vi "PDE_Check Tridiag Solver Platform.vi"(8 "error in (no error)":errorcluster) -> (0 "error out":errorcluster)   [LabVIEW 2017, in "NI_PDE.lvlib"]
uses:
  <vilib>/gmath/NI_PDE.lvlib
  <vilib>/Analysis/NI_AALPro.lvlib
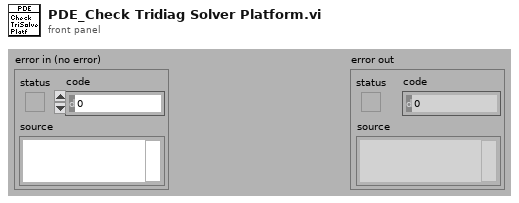
[diagram p1: front panel]
types:
  T1 = cluster{"Diagonal":dbl[], "Super Diagonal":dbl[], "2nd Super Diagonal":dbl[]}
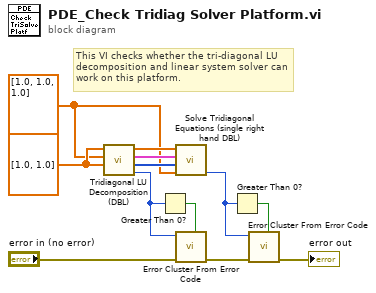
[diagram p0: block diagram]
diagram:
  w7 = dbl[] [1.0, 1.0, 1.0] ("Sub Diagonal")
  w12 = dbl[] [1.0, 1.0] ("Sub Diagonal")
  # "This VI checks whether the tri-diagonal LU decomposition and linear system solver can work on this platform."
  n1 = call <vilib>:"Tridiagonal LU Decomposition (DBL).vi"("Super Diagonal"=w12, "Diagonal"=w7, "Sub Diagonal"=w12) -> ("error"=w4:i32, "Pivot"=w8:i32[], "U"=w9:T1, "L"=w10:dbl[])  [unwired: 5 out]
  n2 = Greater Than 0?(x=w4) -> (x > 0?=w6:bool)
  n3 = call <vilib>:"Solve Tridiagonal Equations (single right hand DBL).vi"("Known Vector"=w7, "Pivot"=w8, "U"=w9, "L"=w10) -> ("error"=w5:i32)  [unwired: 7 out]
  n4 = call <vilib>:"Error Cluster From Error Code.vi"("is warning? (False)"=w6, "error in (no error)"="error in (no error)", "error code (0)"=w4) -> ("error out"=w2:errorcluster)  [unwired: 1 in, 5 out]
  n5 = Greater Than 0?(x=w5) -> (x > 0?=w11:bool)
  n6 = call <vilib>:"Error Cluster From Error Code.vi"("is warning? (False)"=w11, "error in (no error)"=w2, "error code (0)"=w5) -> ("error out"=→"error out":errorcluster)  [unwired: 1 in, 5 out]
